vi "rt_auto_disp_2.vi"(2 "LightProbability":u32, 3 "Mean":dbl=1.0, 4 "Enable":bool) -> (0 "OptoChanceOnArray":bool[](array[boolean]), 1 "Dispense":bool)   [LabVIEW 2013]
uses:
  <vilib>/gmath/statdist.llb/Uniform (Discrete) Random.vi
  <vilib>/gmath/statdist.llb/Poisson Random.vi
  <vilib>/gmath/NI_Gmath.lvlib
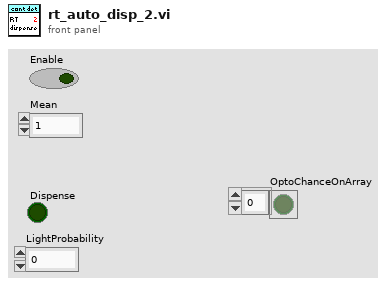
[diagram p1: front panel]
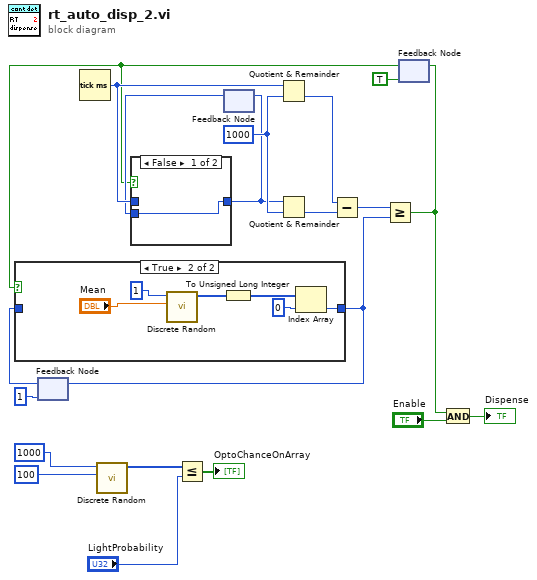
[diagram p0: block diagram]
diagram:
  w11 = u32 1000 ("y")
  n1 = feedback #1(u32 1 ("Numeric")) -> (w10:u32)
  n2 = Tick Count (ms)() -> (millisecond timer value=w20:u32)
  n3 = call-poly <vilib>:"Discrete Random.vi"("n"=100, "samples"=1000) -> ("uniform (discrete) random data"=w2:i32[])  [unwired: 8 in, 1 out]
  n4 = Less Or Equal?(x=w2, y="LightProbability") -> (x <= y?=→"OptoChanceOnArray":bool[])
  n5 = feedback #2() -> (w16:u32)  [unwired: 1 in]
  n6 = Quotient & Remainder(x=w20, y=w11) -> (floor(x/y)=w18:u32)  [unwired: 1 out]
  n7 = feedback #3(TRUE) -> (w14:bool)
  n8 = case shown="True" w14 {
    tunnel: [w21 w22] -> w13
    tunnel: w10 -> [w21 _]
    frame False {
    }
    frame True {
      n9 = call-poly <vilib>:"Discrete Random.vi"("lambda"="Mean", "samples"=1) -> ("Poisson random data"=w24:i32[])  [unwired: 8 in, 1 out]
      n10 = To Unsigned Long Integer(number=w24) -> (unsigned 32bit integer=w23:u32[])
      n11 = Index Array(array=w23, index=0) -> (element=w22:u32)
    }
  }
  n12 = feedback-in #1(w13) -> ()
  n13 = case shown="False" w14 {
    tunnel: [w28 w29] -> w6
    tunnel: w20 -> [_ w29]
    tunnel: w16 -> [w28 _]
    frame False {
    }
    frame True {
    }
  }
  n14 = feedback-in #2(w6) -> ()
  n15 = Quotient & Remainder(x=w6, y=w11) -> (floor(x/y)=w12:u32)  [unwired: 1 out]
  n16 = Subtract(x=w18, y=w12) -> (x-y=w19:u32)
  n17 = Greater Or Equal?(x=w19, y=w13) -> (x >= y?=w15:bool)
  n18 = feedback-in #3(w15) -> ()
  n19 = And(x=w15, y="Enable") -> (x .and. y?=→"Dispense":bool)
